vi "go to leaf for traverse.vi"(8 "error in":errorcluster caption="错误输入（无错误）", 10 "Data in":T2, 11 "Class in":refnum<class "PanelLinkNode.lvclass"> caption="DNL_LabVIEW Object in") -> (0 "error out":errorcluster caption="错误输出", 1 "Stop Traverse":bool, 2 "Data out":T1, 3 "Class out":refnum<class "PanelLinkNode.lvclass"> caption="DNL_LabVIEW Object out")   [LabVIEW 2016, in "PanelLinkNode.lvclass"]
uses:
  PanelLinkNode.lvclass
  PanelObject/PanelObject.lvclass
  PanelLinkNode.lvclass/PanelLinkNode.ctl
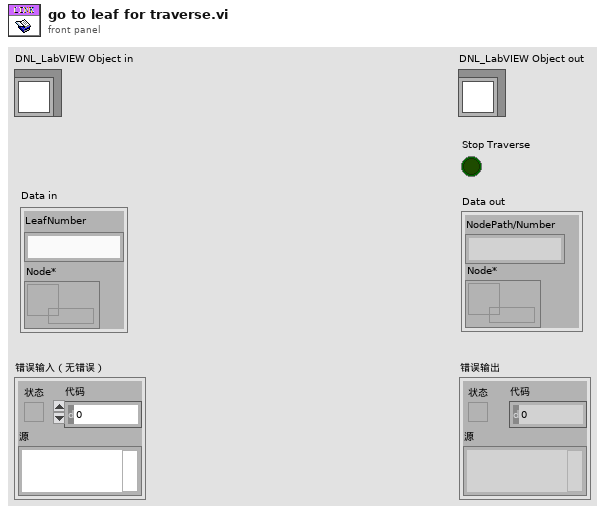
[diagram p1: front panel]
types:
  T1 = cluster{"NodePath/Number":string, "Node*":refnum<data-value>}
  T2 = cluster{"LeafNumber":string, "Node*":refnum<data-value>}
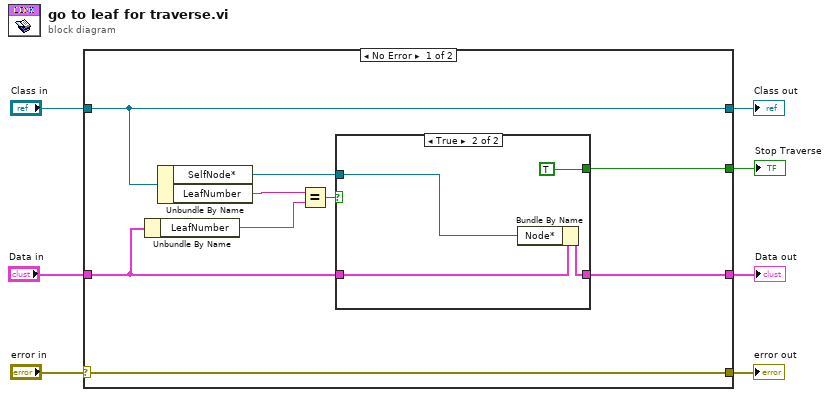
[diagram p0: block diagram]
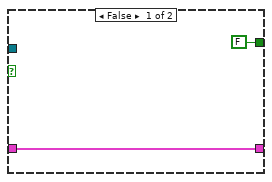
[diagram p2: hidden frame]
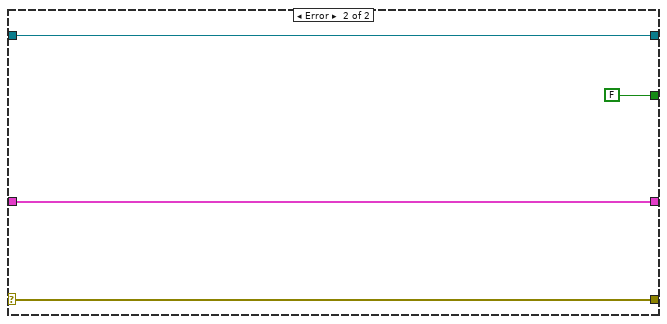
[diagram p3: hidden frame]
diagram:
  n1 = case shown="No Error" "error in" {
    selector: "error in" -> [w16 w26]
    tunnel: [w16 w26] -> w6
    tunnel: [w15 w25] -> w4
    tunnel: "Class in" -> [w15 w25]
    tunnel: "Data in" -> [w11 w24]
    tunnel: [w9 w24] -> w2
    tunnel: [w8 FALSE] -> w1
    frame No Error {
      n2 = Unbundle By Name(w11) -> ("LeafNumber"=w13:string)
      n3 = Unbundle By Name(w15) -> ("SelfNode*"=w10:refnum<data-value>, "LeafNumber"=w14:string)
      n4 = Equal?(x=w14, y=w13) -> (x = y?=w12:bool)
      n5 = case shown="True" w12 {
        tunnel: w11 -> [w18 w22]
        tunnel: w10 -> [_ w20]
        tunnel: [w18 w21] -> w9
        tunnel: [FALSE TRUE] -> w8
        frame False {
        }
        frame True {
          n6 = Bundle By Name(cluster=w22, "Node*"=w20) -> (w21:T2)
        }
      }
    }
    frame Error {
    }
  }
  "error out" <- w6
  "Class out" <- w4
  "Data out" <- w2
  "Stop Traverse" <- w1
